vi "To Lower.vi"(4 "String":refnum<class "Abs_String.lvclass">) -> (1 "Result":refnum<class "Abs_String.lvclass">)   [LabVIEW 2021]
uses:
  Abs_Types/String/Abs_String.lvclass
  Support/ToLower/ToLower_STR.lvclass
  C:/TSA/LV_Abstract/Source/Functions/Support/Function/One Terminal/STR/AbsFunc_One Term_STR.lvclass
  C:/Program Files (x86)/National Instruments/LabVIEW 2021/vi.lib/TSA/Abstract Data Classes/Abs_Types/String/Abs_String.lvclass
  Support/Function/One Terminal/STR/AbsFunc_One Term_STR.lvclass/AbsFunc_One Term_STR.ctl
  Support/Function/One Terminal/STR/Properties/Write String A.vi
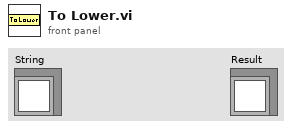
[diagram p1: front panel]
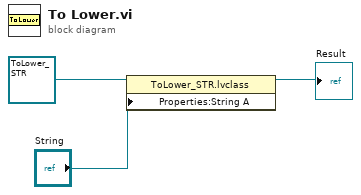
[diagram p0: block diagram]
diagram:
  n1 = property class="ToLower_STR.lvclass"(reference=refnum<class "ToLower_STR.lvclass"> refnum ("ToLower_STR.lvclass"), "Properties:String A"="String") -> (reference out=→"Result":refnum<class "ToLower_STR.lvclass">)  [unwired: 1 in, 1 out]
